vi "Teleop.vi"(0 "Call Context":T10) -> (6 "SubState 3":T1, 8 "SubState 4":T1, 9 "SubState 5":T9, 11 "Loop 3 Data":T5, 13 "Loop 4 Data":T4, 14 "SubState 0":T1=enum."driver control", 15 "Loop 1 Data":T7, 16 "Loop 0 Data":T8, 17 "SubState 1":T1, 18 "Loop 2 Data":T6, 19 "SubState 2":T1)   [LabVIEW 2013]
uses:
  typedefs/subStates.ctl
  <vilib>/Rock Robotics/WPI/DriverStation/WPI_DriverStationDerivedRobotMode.ctl
  typedefs/singleUseSubstate.ctl
  typedefs/Loop Datatypes/Loop 0 Datatype.ctl
  typedefs/Loop Datatypes/Loop 1 Datatype.ctl
  typedefs/Loop Datatypes/Loop 2 Datatype.ctl
  typedefs/Loop Datatypes/Loop 3 Datatype.ctl
  typedefs/Loop Datatypes/Loop 4 Datatype.ctl
  <vilib>/Rock Robotics/WPI/Joystick/WPI_JoystickDevRef.ctl
  <vilib>/Rock Robotics/WPI/Joystick/WPI_JoystickDeviceEnum.ctl
  typedefs/fg_typedef.ctl
  typedefs/vision enable.ctl
  <vilib>/Rock Robotics/WPI/Joystick/WPI_JoystickGetSetRefNum.vi
panel:
  out "prev lock state":T1
  out "JS3":T2
  out "Drive to DC":bool
  out "JS1":T2
  out "JS2":T2
  out "Exit Value":i32=-1
  # "Loop Data and Substates"
  # "Latch Loop"
  # "Drive Loop"
  # "Shooter Pneumatics Loop"
  # "Pickup/Passing Belts Loop"
  # "Pickup Arm Loop"
  # "Shifter Loop"
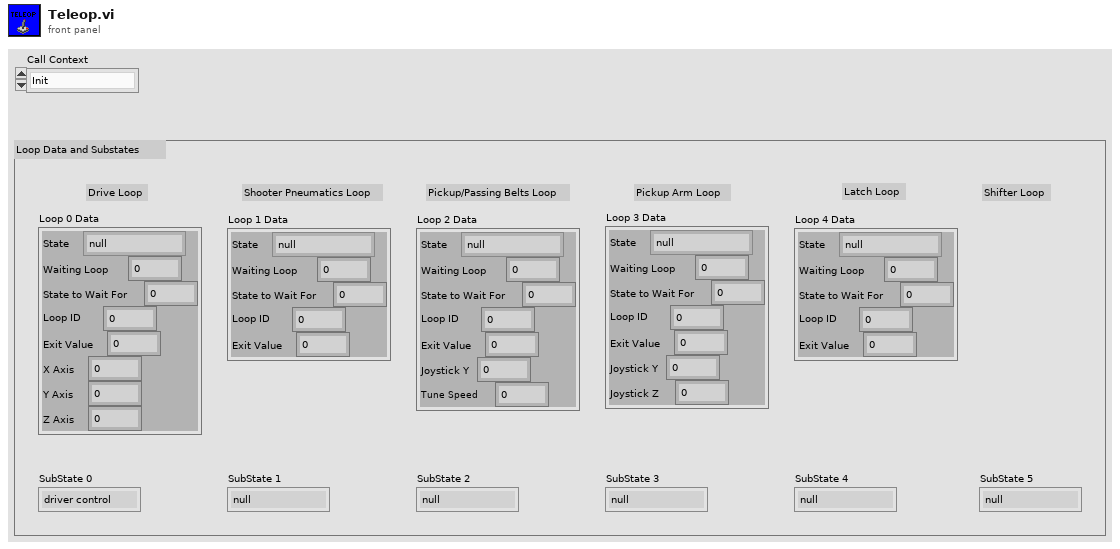
[diagram p1: front panel]
types:
  T1 = typedef "subStates.ctl" = enum16{"null", "wait", "driver control", "auto", "manual override", "hold position", "rotate", "pickup", "pass", "load", "goto shoot", "shoot", "cancel", "end"}
  T2 = typedef "WPI_JoystickDevRef.ctl" = cluster{"Device":T3}
  T3 = typedef "WPI_JoystickDeviceEnum.ctl" = enum16{"USB 1", "USB 2", "USB 3", "USB 4", "Kinect 1", "Kinect 2"}
  T4 = typedef "Loop 4 Datatype.ctl" = cluster{"State":T1, "Waiting Loop":i32, "State to Wait For":i32, "Loop ID":i32, "Exit Value":i32}
  T5 = typedef "Loop 3 Datatype.ctl" = cluster{"State":T1, "Waiting Loop":i32, "State to Wait For":i32, "Loop ID":i32, "Exit Value":i32, "Joystick Y":dbl, "Joystick Z":dbl}
  T6 = typedef "Loop 2 Datatype.ctl" = cluster{"State":T1, "Waiting Loop":i32, "State to Wait For":i32, "Loop ID":i32, "Exit Value":i32, "Joystick Y":dbl, "Tune Speed":dbl}
  T7 = typedef "Loop 1 Datatype.ctl" = cluster{"State":T1, "Waiting Loop":i32, "State to Wait For":i32, "Loop ID":i32, "Exit Value":i32}
  T8 = typedef "Loop 0 Datatype.ctl" = cluster{"State":T1, "Waiting Loop":i32, "State to Wait For":i32, "Loop ID":i32, "Exit Value":i32, "X Axis":dbl, "Y Axis":dbl, "Z Axis":dbl}
  T9 = typedef "singleUseSubstate.ctl" = enum16{"null", "wait", "shift high", "shift low", "extend shooter", "retract shooter", "close latch", "open latch"}
  T10 = typedef "WPI_DriverStationDerivedRobotMode.ctl" = enum16{"Init", "Execute", "Stop"}
  T11 = cluster{"axis 1 (x)":dbl, "axis 2 (y)":dbl, "axis 3 (throttle)":dbl, "axis 4":dbl, "axis 5":dbl, "axis 6":dbl}
  T12 = typedef "WPI_EncoderDevRef.ctl" = cluster{"DevStatus":errorcluster, "EncoderIndex":T13, "CounterIndex":T14, "DistancePerCount":dbl, "Decoding Type":T15}
  T13 = typedef "FPGA_EncoderIdx.ctl" = enum8{"Enc 0", "Enc 1", "Enc 2", "Enc 3", "Invalid"}
  T14 = typedef "FPGA_CounterCtrSystemIndex.ctl" = enum8{"Ctr 0", "Ctr 1", "Ctr 2", "Ctr 3", "Ctr 4", "Ctr 5", "Ctr 6", "Ctr 7", "Invalid"}
  T15 = typedef "WPI_EncoderType.ctl" = enum16{"1x", "2x", "4x"}
  T16 = typedef "vision enable.ctl" = enum16{"Enable", "Disable", "Stop"}
  T17 = typedef "fg_typedef.ctl" = enum16{"Get", "Set"}
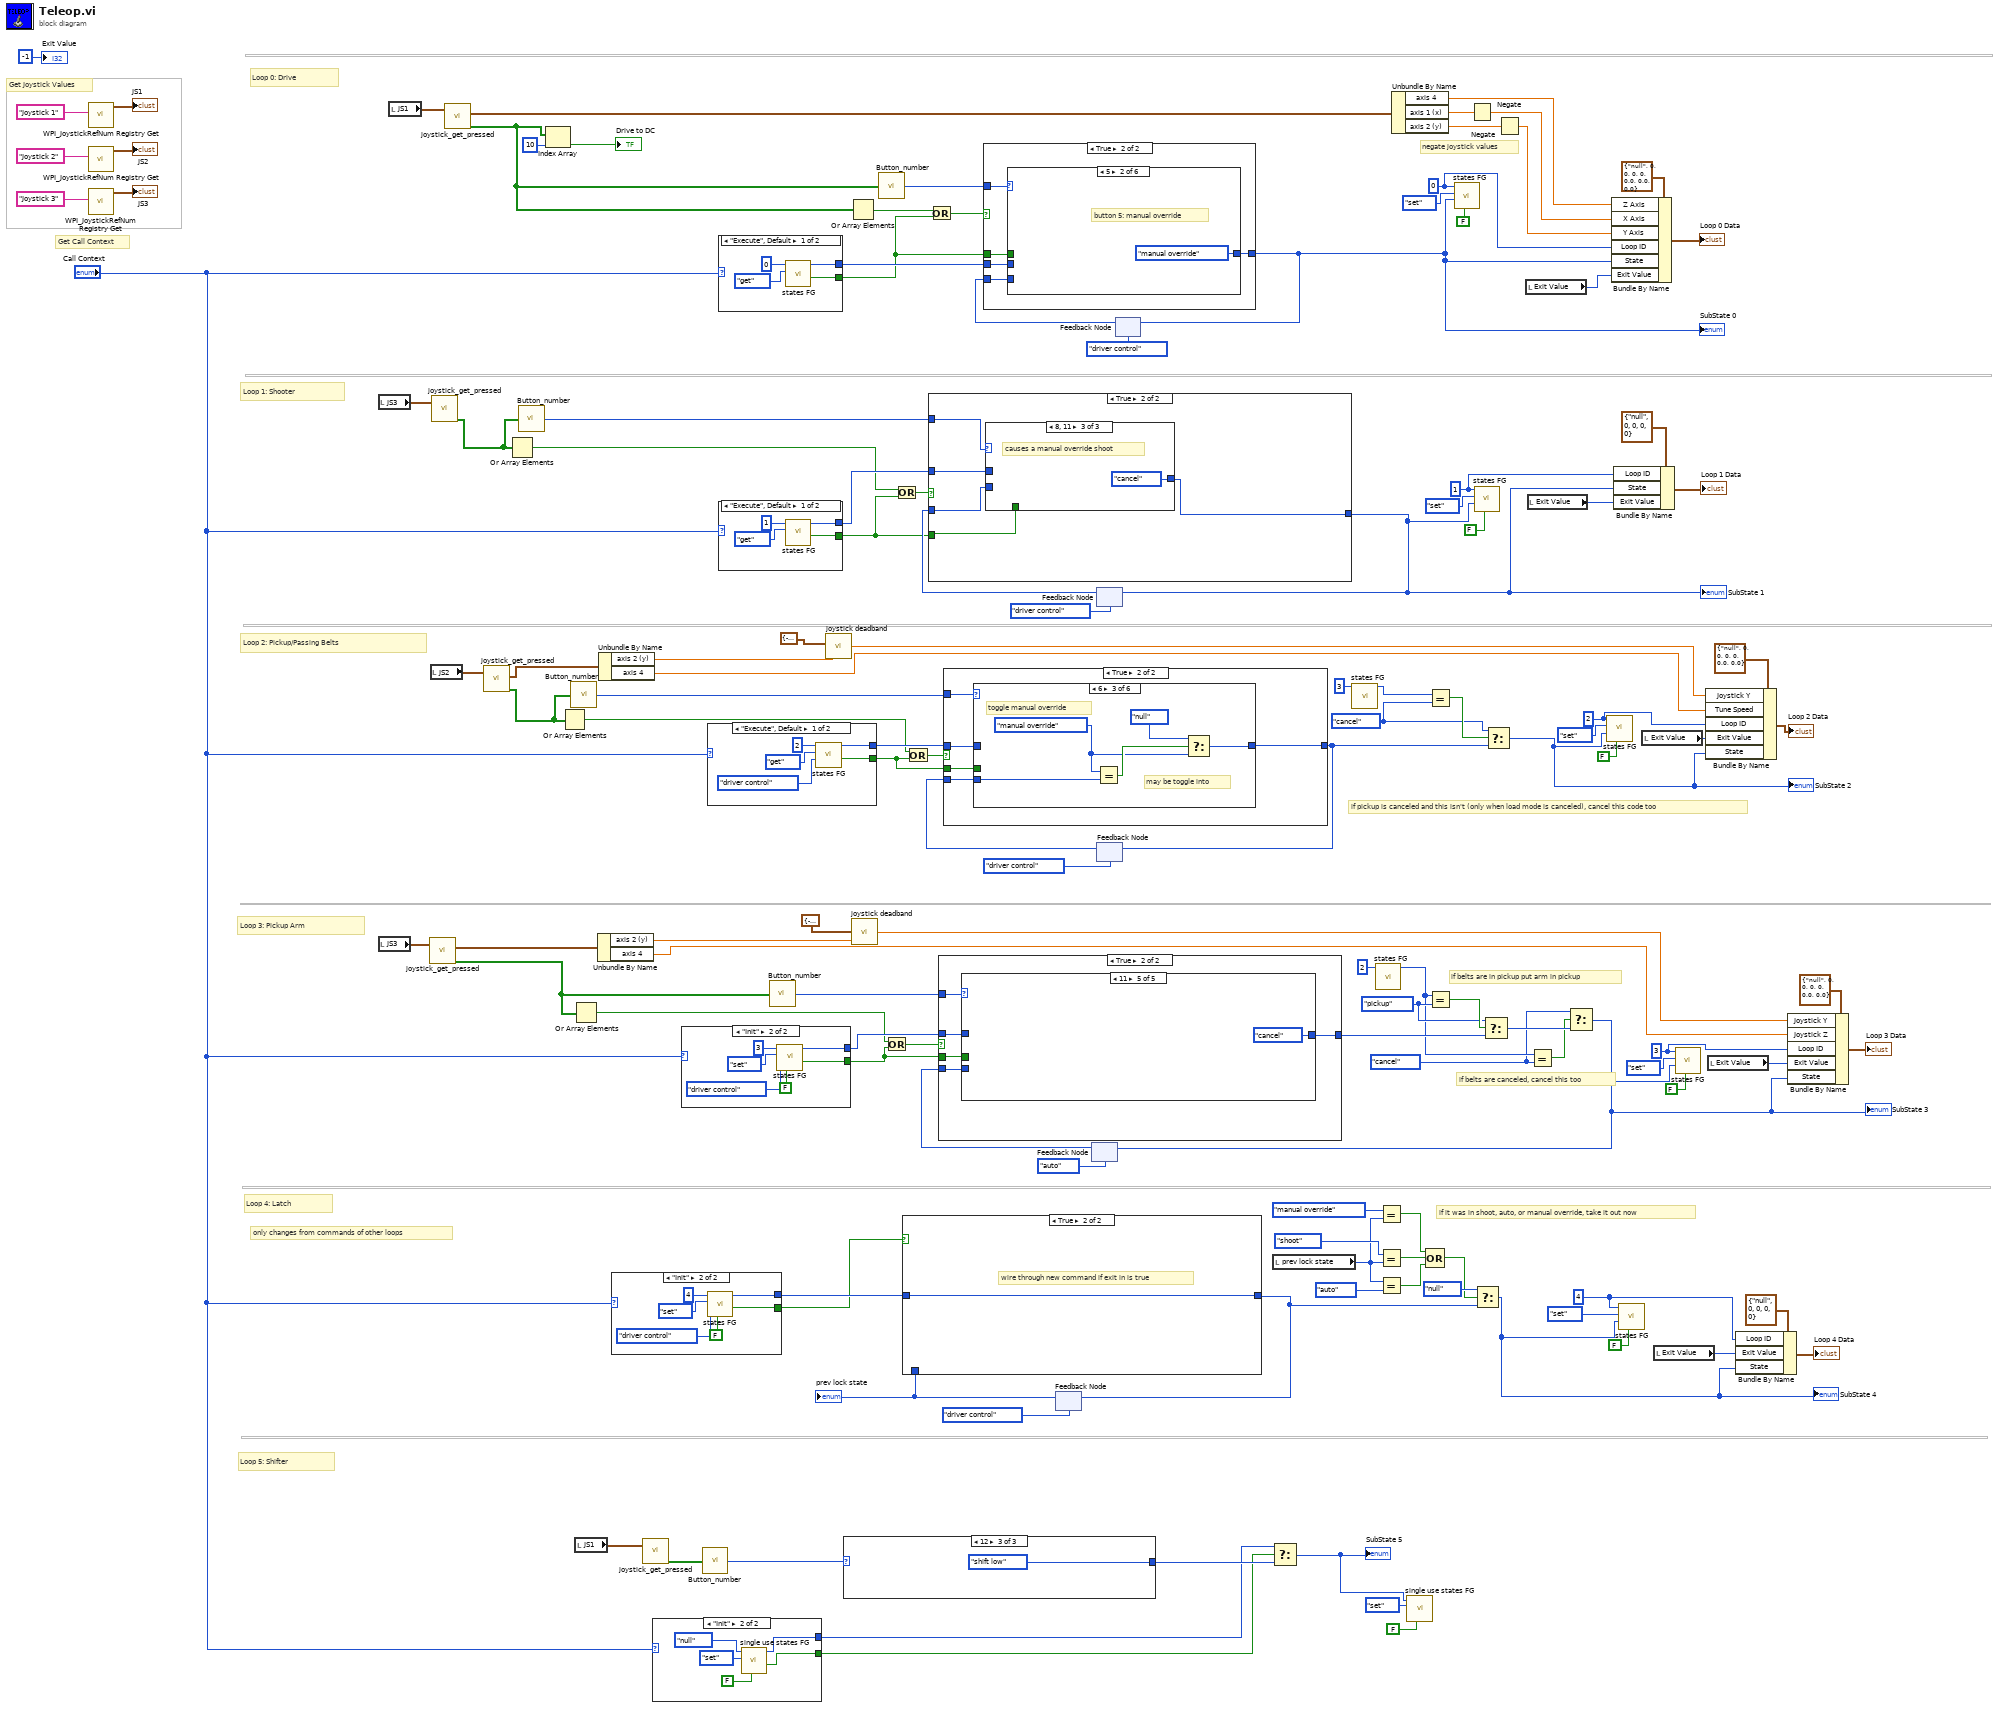
[diagram p0: block diagram]
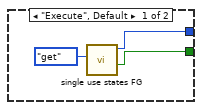
[diagram p2: hidden frame]
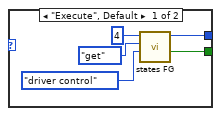
[diagram p4: hidden frame]
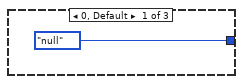
[diagram p5: hidden frame]
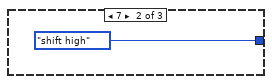
[diagram p6: hidden frame]
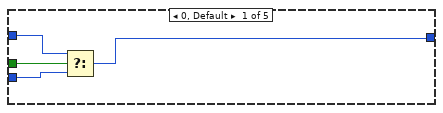
[diagram p8: hidden frame]
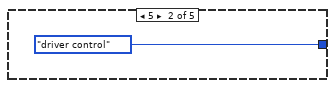
[diagram p9: hidden frame]
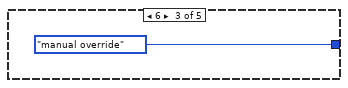
[diagram p10: hidden frame]
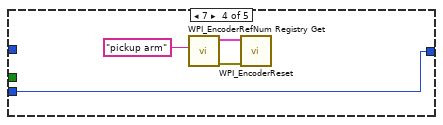
[diagram p11: hidden frame]
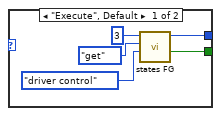
[diagram p12: hidden frame]
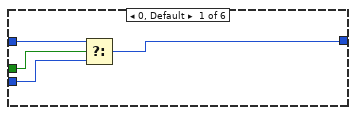
[diagram p14: hidden frame]
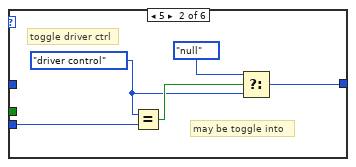
[diagram p15: hidden frame]
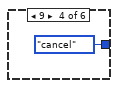
[diagram p16: hidden frame]
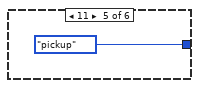
[diagram p17: hidden frame]
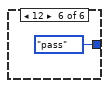
[diagram p18: hidden frame]
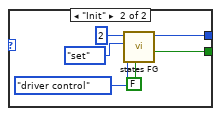
[diagram p19: hidden frame]
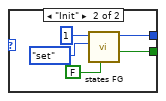
[diagram p20: hidden frame]
diagram:
  w7 = subStates."cancel" ("y")
  w14 = subStates."cancel" ("y")
  w31 = subStates."pickup" ("y")
  w42 = 4 ("Loop ID")
  w105 = 3 ("Loop ID")
  w106 = 2 ("Loop ID")
  w115 = 1 ("Loop ID")
  w117 = 0 ("Loop ID")
  # "if pickup is canceled and this isn't (only when load mode is canceled), cancel this code too"
  # "if belts are canceled, cancel this too"
  # "only changes from commands of other loops"
  # "if it was in shoot, auto, or manual override, take it out now"
  # "if belts are in pickup put arm in pickup"
  # "negate joystick values"
  # "Get Call Context"
  # "Get Joystick Values"
  # "Loop 4: Latch"
  # "Loop 3: Pickup Arm"
  # "Loop 5: Shifter"
  # "Loop 2: Pickup/Passing Belts"
  # "Loop 1: Shooter"
  # "Loop 0: Drive"
  n1 = call <vilib>:"WPI_JoystickRefNum Registry Get.vi"("refnum name"="Joystick 1") -> ("JoystickDevRef"=→"JS1":T2)  [unwired: 9 in, 1 out]
  n2 = call <vilib>:"WPI_JoystickRefNum Registry Get.vi"("refnum name"="Joystick 2") -> ("JoystickDevRef"=→"JS2":T2)  [unwired: 9 in, 1 out]
  n3 = call <vilib>:"WPI_JoystickRefNum Registry Get.vi"("refnum name"="Joystick 3") -> ("JoystickDevRef"=→"JS3":T2)  [unwired: 9 in, 1 out]
  n4 = local read "JS3"() -> (w82:T2)
  n5 = local read "JS3"() -> (w67:T2)
  n6 = local read "JS1"() -> (w83:T2)
  n7 = call "joystick_get_pressed.vi"("JoystickDevRef 2"=w67) -> ("Axes"=w71:T11, "Buttons Pressed?"=w49:bool[])  [unwired: 1 in, 2 out]
  n8 = local read "JS2"() -> (w56:T2)
  n9 = call "joystick_get_pressed.vi"("JoystickDevRef 2"=w82) -> ("Buttons Pressed?"=w51:bool[])  [unwired: 1 in, 3 out]
  n10 = call "joystick_get_pressed.vi"("JoystickDevRef 2"=w83) -> ("Axes"=w87:T11, "Buttons Pressed?"=w63:bool[])  [unwired: 1 in, 2 out]
  n11 = call "joystick_get_pressed.vi"("JoystickDevRef 2"=w56) -> ("Axes"=w39:T11, "Buttons Pressed?"=w40:bool[])  [unwired: 1 in, 2 out]
  n12 = Or Array Elements(Boolean array=w51) -> (logical OR=w74:bool)
  n13 = call "Button_number.vi"("Button Array"=w51) -> ("Button Pressed"=w76:i32)
  n14 = Index Array(array=w63, index=10) -> (element=→"Drive to DC":bool)
  n15 = Or Array Elements(Boolean array=w40) -> (logical OR=w55:bool)
  n16 = call "Button_number.vi"("Button Array"=w40) -> ("Button Pressed"=w54:i32)
  n17 = Or Array Elements(Boolean array=w49) -> (logical OR=w70:bool)
  n18 = local read "JS1"() -> (w59:T2)
  n19 = Unbundle By Name(w71) -> ("axis 2 (y)"=w66:dbl, "axis 4"=w35:dbl)
  n20 = Unbundle By Name(w39) -> ("axis 2 (y)"=w48:dbl, "axis 4"=w37:dbl)
  n21 = case shown="\"Init\"" "Call Context" {
    tunnel: [w136 w142] -> w19
    tunnel: [w134 w139] -> w44
    frame "Execute", Default {
      n22 = call "states FG.vi"("subState in"=subStates."driver control", "menu (get)"=enum16{"set", "get"}."get", "Loop ID"=4) -> ("exit out"=w136:bool, "subState out"=w134:T1)  [unwired: 5 in, 2 out]
    }
    frame "Init" {
      n23 = call "states FG.vi"("exit in"=FALSE, "subState in"=subStates."driver control", "menu (get)"=enum16{"set", "get"}."set", "Loop ID"=4) -> ("exit out"=w142:bool, "subState out"=w139:T1)  [unwired: 4 in, 2 out]
    }
  }
  n24 = call "joystick_get_pressed.vi"("JoystickDevRef 2"=w59) -> ("Buttons Pressed?"=w61:bool[])  [unwired: 1 in, 3 out]
  n25 = case shown="\"Init\"" "Call Context" {
    tunnel: [w146 w148] -> w4
    tunnel: [w145 w149] -> w5
    frame "Execute", Default {
      n26 = call "single use states FG.vi"("menu (get)"=enum16{"set", "get"}."get") -> ("exit out"=w146:bool, "substate out"=w145:T9)  [unwired: 7 in, 2 out]
    }
    frame "Init" {
      n27 = call "single use states FG.vi"("exit in"=FALSE, "menu (get)"=enum16{"set", "get"}."set", "substate"=singleUseSubstate."null") -> ("exit out"=w148:bool, "substate out"=w149:T9)  [unwired: 5 in, 2 out]
    }
  }
  n28 = case shown="\"Init\"" "Call Context" {
    tunnel: [w155 w161] -> w68
    tunnel: [w153 w158] -> w103
    frame "Execute", Default {
      n29 = call "states FG.vi"("subState in"=subStates."driver control", "menu (get)"=enum16{"set", "get"}."get", "Loop ID"=3) -> ("exit out"=w155:bool, "subState out"=w153:T1)  [unwired: 5 in, 2 out]
    }
    frame "Init" {
      n30 = call "states FG.vi"("exit in"=FALSE, "subState in"=subStates."driver control", "menu (get)"=enum16{"set", "get"}."set", "Loop ID"=3) -> ("exit out"=w161:bool, "subState out"=w158:T1)  [unwired: 4 in, 2 out]
    }
  }
  n31 = call "Button_number.vi"("Button Array"=w61) -> ("Button Pressed"=w60:i32)
  n32 = case shown="\"Execute\", Default" "Call Context" {
    tunnel: [w166 w172] -> w73
    tunnel: [w164 w169] -> w122
    frame "Execute", Default {
      n33 = call "states FG.vi"("subState in"=subStates."driver control", "menu (get)"=enum16{"set", "get"}."get", "Loop ID"=2) -> ("exit out"=w166:bool, "subState out"=w164:T1)  [unwired: 5 in, 2 out]
    }
    frame "Init" {
      n34 = call "states FG.vi"("exit in"=FALSE, "subState in"=subStates."driver control", "menu (get)"=enum16{"set", "get"}."set", "Loop ID"=2) -> ("exit out"=w172:bool, "subState out"=w169:T1)  [unwired: 4 in, 2 out]
    }
  }
  n35 = case shown="\"Execute\", Default" "Call Context" {
    tunnel: [w176 w181] -> w80
    tunnel: [w175 w179] -> w120
    frame "Execute", Default {
      n36 = call "states FG.vi"("menu (get)"=enum16{"set", "get"}."get", "Loop ID"=0) -> ("exit out"=w176:bool, "subState out"=w175:T1)  [unwired: 6 in, 2 out]
    }
    frame "Init" {
      n37 = call "states FG.vi"("exit in"=FALSE, "menu (get)"=enum16{"set", "get"}."set", "Loop ID"=0) -> ("exit out"=w181:bool, "subState out"=w179:T1)  [unwired: 5 in, 2 out]
    }
  }
  n38 = case shown="\"Execute\", Default" "Call Context" {
    tunnel: [w185 w190] -> w77
    tunnel: [w184 w188] -> w119
    frame "Execute", Default {
      n39 = call "states FG.vi"("menu (get)"=enum16{"set", "get"}."get", "Loop ID"=1) -> ("exit out"=w185:bool, "subState out"=w184:T1)  [unwired: 6 in, 2 out]
    }
    frame "Init" {
      n40 = call "states FG.vi"("exit in"=FALSE, "menu (get)"=enum16{"set", "get"}."set", "Loop ID"=1) -> ("exit out"=w190:bool, "subState out"=w188:T1)  [unwired: 5 in, 2 out]
    }
  }
  n41 = call "Button_number.vi"("Button Array"=w49) -> ("Button Pressed"=w69:i32)
  n42 = call "joystick deadband.vi"("Joystick In"=w48, "Deadband Range"=cluster{"Deadband Min":dbl, "Deadband Max":dbl} {"Deadband Min"=-0.05, "Deadband Max"=0.05}) -> ("Joystick Out"=w38:dbl)  [unwired: 4 in]
  n43 = case shown="12" w60 {
    tunnel: [singleUseSubstate."null" ("Enum") singleUseSubstate."shift high" ("Enum") singleUseSubstate."shift low" ("Enum")] -> w95
    frame 0, Default {
    }
    frame 7 {
    }
    frame 12 {
    }
  }
  n44 = Or Array Elements(Boolean array=w63) -> (logical OR=w81:bool)
  n45 = call "joystick deadband.vi"("Joystick In"=w66, "Deadband Range"=cluster{"Deadband Min":dbl, "Deadband Max":dbl} {"Deadband Min"=-0.05, "Deadband Max"=0.05}) -> ("Joystick Out"=w36:dbl)  [unwired: 4 in]
  n46 = call "Button_number.vi"("Button Array"=w63) -> ("Button Pressed"=w86:i32)
  n47 = Or(x=w70, y=w68) -> (x .or. y?=w72:bool)
  n48 = Or(x=w74, y=w77) -> (x .or. y?=w78:bool)
  n49 = Or(x=w55, y=w73) -> (x .or. y?=w75:bool)
  n50 = Or(x=w81, y=w80) -> (x .or. y?=w79:bool)
  n51 = feedback #1(subStates."driver control" ("Drive SubState")) -> (w18:T1)
  "prev lock state" <- w18
  n52 = case shown="True" w19 {
    tunnel: [w196 w197] -> w29
    tunnel: w44 -> [_ w197]
    tunnel: w18 -> [w196 _]
    frame False {
      # "*yawn* nothing to do...wire through the previous state"
    }
    frame True {
      # "wire through new command if exit in is true"
    }
  }
  n53 = feedback-in #1(w29) -> ()
  n54 = feedback #2(subStates."auto" ("Drive SubState")) -> (w100:T1)
  n55 = case shown="True" w72 {
    tunnel: w100 -> [w198 w199]
    tunnel: [w198 w200] -> w33
    tunnel: w103 -> [_ w201]
    tunnel: w69 -> [_ w203]
    tunnel: w68 -> [_ w202]
    frame False {
      # "boring drivers, not pressing anything...wire through the previous state"
    }
    frame True {
      n56 = case shown="11" w203 {
        tunnel: w202 -> [w207 _ _ _ _]
        tunnel: w199 -> [w206 _ _ w213 _]
        tunnel: w201 -> [w205 _ _ _ _]
        tunnel: [w204 subStates."driver control" ("Drive SubState") subStates."manual override" ("Drive SubState") w213 subStates."cancel" ("Drive SubState")] -> w200
        frame 0, Default {
          n57 = Select(t=w205, s=w207, f=w206) -> (s? t:f=w204:T1)
        }
        frame 5 {
        }
        frame 6 {
        }
        frame 7 {
          n58 = call <vilib>:"WPI_EncoderRefNum Registry Get.vi"("refnum name"="pickup arm") -> ("error out"=w211:errorcluster, "EncoderDevRef"=w210:T12)  [unwired: 9 in]
          n59 = call <vilib>:"WPI_EncoderReset.vi"("error in (no error)"=w211, "EncoderDevRef"=w210) -> ()  [unwired: 8 in, 2 out]
        }
        frame 11 {
        }
      }
    }
  }
  n60 = feedback #3(subStates."driver control" ("Drive SubState")) -> (w121:T1)
  n61 = case shown="True" w78 {
    tunnel: w121 -> [w215 w219]
    tunnel: [w215 w216] -> w88
    tunnel: w119 -> [_ w220]
    tunnel: w76 -> [_ w218]
    tunnel: w77 -> [_ w217]
    frame False {
      # "nothing pressed here, move along (wire through the previous state)"
    }
    frame True {
      n62 = case shown="8, 11" w218 {
        tunnel: w220 -> [w223 _ _]
        tunnel: w219 -> [w222 _ _]
        tunnel: [w221 subStates."load" ("Drive SubState") subStates."cancel" ("Drive SubState")] -> w216
        tunnel: w217 -> [w224 _ _]
        frame 0, Default {
          n63 = Select(t=w223, s=w224, f=w222) -> (s? t:f=w221:T1)
        }
        frame 2 {
        }
        frame 8, 11 {
          # "causes a manual override shoot"
        }
      }
    }
  }
  "SubState 1" <- w88
  n64 = feedback-in #3(w88) -> ()
  n65 = feedback #4(subStates."driver control" ("Drive SubState")) -> (w125:T1)
  n66 = case shown="True" w75 {
    tunnel: w125 -> [w227 w229]
    tunnel: [w227 w228] -> w10
    tunnel: w122 -> [_ w230]
    tunnel: w54 -> [_ w232]
    tunnel: w73 -> [_ w231]
    frame False {
      # "nothing pressed here, move along obviously and wire through the previous state"
    }
    frame True {
      n67 = case shown="6" w232 {
        tunnel: w231 -> [w236 _ _ _ _ _]
        tunnel: w230 -> [w235 _ _ _ _ _]
        tunnel: w229 -> [w234 w241 w243 _ _ _]
        tunnel: [w233 w237 w242 subStates."cancel" ("Drive SubState") subStates."pickup" ("Drive SubState") subStates."pass" ("Drive SubState")] -> w228
        frame 0, Default {
          n68 = Select(t=w235, s=w236, f=w234) -> (s? t:f=w233:T1)
        }
        frame 5 {
          w239 = subStates."driver control" ("Drive SubState")
          # "may be toggle into"
          # "toggle driver ctrl"
          n69 = Equal?(x=w239, y=w241) -> (x = y?=w240:bool)
          n70 = Select(t=subStates."null", s=w240, f=w239) -> (s? t:f=w237:T1)
        }
        frame 6 {
          w244 = subStates."manual override" ("Drive SubState")
          # "may be toggle into"
          # "toggle manual override"
          n71 = Equal?(x=w244, y=w243) -> (x = y?=w246:bool)
          n72 = Select(t=subStates."null", s=w246, f=w244) -> (s? t:f=w242:T1)
        }
        frame 9 {
        }
        frame 11 {
        }
        frame 12 {
        }
      }
    }
  }
  n73 = feedback-in #4(w10) -> ()
  n74 = feedback #5(subStates."driver control" ("Drive SubState")) -> (w127:T1)
  n75 = case shown="True" w79 {
    tunnel: w127 -> [w250 w252]
    tunnel: [w250 w251] -> w58
    tunnel: w120 -> [_ w253]
    tunnel: w86 -> [_ w255]
    tunnel: w80 -> [_ w254]
    frame False {
      # "keep current state, no change necessary"
    }
    frame True {
      n76 = case shown="5" w255 {
        tunnel: w254 -> [w259 _ _ _ _ _]
        tunnel: w253 -> [w258 _ _ _ _ _]
        tunnel: w252 -> [w257 _ w265 w266 w274 _]
        tunnel: [w256 subStates."manual override" ("Drive SubState") w261 w266 w275 subStates."driver control" ("Drive SubState")] -> w251
        frame 0, Default {
          n77 = Select(t=w258, s=w259, f=w257) -> (s? t:f=w256:T1)
        }
        frame 5 {
          # "button 5: manual override"
        }
        frame 1 {
          w262 = subStates."hold position" ("x")
          # "button 1, hold position toggle"
          n78 = Equal?(x=w262, y=w265) -> (x = y?=w264:bool)
          n79 = Select(t=subStates."driver control" ("Drive SubState"), s=w264, f=w262) -> (s? t:f=w261:T1)
        }
        frame 8 {
          n80 = disable-structure shown="Enabled" {
            frame Disabled {
              w269 = vision_enable."Enable" ("y")
              # "toggle vision"
              n81 = call "vision_fg.vi"("Menu"=fg_typedef."Get") -> ("State Out"=w271:T16)  [unwired: 2 in, 1 out]
              n82 = Equal?(x=w271, y=w269) -> (x = y?=w270:bool)
              n83 = Select(t=vision_enable."Disable" ("y"), s=w270, f=w269) -> (s? t:f=w267:T16)
              n84 = call "vision_fg.vi"("Action"=w267, "Menu"=fg_typedef."Set") -> ()  [unwired: 1 in, 2 out]
            }
            frame Enabled {
              # "no vision at suffield"
            }
          }
        }
        frame 9 {
          n85 = disable-structure shown="Enabled" {
            disable-tunnel: [subStates."goto shoot" ("Drive SubState") w279] -> w275
            disable-tunnel: w274 -> [_ w279]
            frame Disabled {
              # "go to shoot location"
              n86 = call "vision_fg.vi"("Action"=vision_enable."Enable", "Menu"=fg_typedef."Set") -> ()  [unwired: 1 in, 2 out]
            }
            frame Enabled {
              # "no vision at suffield"
            }
          }
        }
        frame 11 {
          # "put robot drive in driver control"
          n87 = call "vision_fg.vi"("Action"=vision_enable."Disable", "Menu"=fg_typedef."Set") -> ()  [unwired: 1 in, 2 out]
        }
      }
    }
  }
  "SubState 0" <- w58
  n88 = feedback-in #5(w58) -> ()
  n89 = Select(t=w5, s=w4, f=w95) -> (s? t:f=w2:T9)
  "SubState 5" <- w2
  n90 = local read "prev lock state"() -> (w25:T1)
  n91 = call "states FG.vi"("Loop ID"=3) -> ("subState out"=w11:T1)  [unwired: 7 in, 3 out]
  n92 = call "states FG.vi"("Loop ID"=2) -> ("subState out"=w17:T1)  [unwired: 7 in, 3 out]
  n93 = Equal?(x=subStates."manual override", y=w25) -> (x = y?=w23:bool)
  n94 = Equal?(x=subStates."shoot", y=w25) -> (x = y?=w22:bool)
  n95 = Equal?(x=w25, y=subStates."auto") -> (x = y?=w21:bool)
  n96 = Unbundle By Name(w87) -> ("axis 4"=w64:dbl, "axis 1 (x)"=w92:dbl, "axis 2 (y)"=w91:dbl)
  n97 = call "single use states FG.vi"("exit in"=FALSE, "menu (get)"=enum16{"set", "get"}."set", "substate"=w2) -> ()  [unwired: 5 in, 4 out]
  n98 = Compound Arithmetic op=OR(w23, w22, w21) -> (w20:bool)
  n99 = Equal?(x=w11, y=w7) -> (x = y?=w9:bool)
  n100 = Equal?(x=w17, y=w31) -> (x = y?=w32:bool)
  n101 = call "states FG.vi"("exit in"=FALSE, "subState in"=w58, "menu (get)"=enum16{"set", "get"}."set", "Loop ID"=w117) -> ()  [unwired: 4 in, 4 out]
  n102 = Negate(x=w92) -> (-x=w90:dbl)
  n103 = call "states FG.vi"("exit in"=FALSE, "subState in"=w88, "menu (get)"=enum16{"set", "get"}."set", "Loop ID"=w115) -> ()  [unwired: 4 in, 4 out]
  n104 = Select(t=subStates."null", s=w20, f=w29) -> (s? t:f=w28:T1)
  "SubState 4" <- w28
  n105 = Select(t=w31, s=w32, f=w33) -> (s? t:f=w16:T1)
  n106 = Select(t=w7, s=w9, f=w10) -> (s? t:f=w8:T1)
  "SubState 2" <- w8
  n107 = Negate(x=w91) -> (-x=w89:dbl)
  n108 = local read "Exit Value"() -> (w113:i32)
  n109 = local read "Exit Value"() -> (w112:i32)
  n110 = Equal?(x=w17, y=w14) -> (x = y?=w15:bool)
  n111 = Select(t=w14, s=w15, f=w16) -> (s? t:f=w13:T1)
  "SubState 3" <- w13
  n112 = feedback-in #2(w13) -> ()
  n113 = call "states FG.vi"("exit in"=FALSE, "subState in"=w8, "menu (get)"=enum16{"set", "get"}."set", "Loop ID"=w106) -> ()  [unwired: 4 in, 4 out]
  n114 = Bundle By Name(cluster=T8 {"State"=enum."null", "Waiting Loop"=0, "State to Wait For"=0, "Loop ID"=0, "Exit Value"=0, "X Axis"=0.0, "Y Axis"=0.0, "Z Axis"=0.0} ("Cluster"), "Z Axis"=w64, "X Axis"=w90, "Y Axis"=w89, "Loop ID"=w117, "State"=w58, "Exit Value"=w113) -> (→"Loop 0 Data":T8)
  n115 = Bundle By Name(cluster=T7 {"State"=enum."null", "Waiting Loop"=0, "State to Wait For"=0, "Loop ID"=0, "Exit Value"=0} ("Cluster"), "Loop ID"=w115, "State"=w88, "Exit Value"=w112) -> (→"Loop 1 Data":T7)
  n116 = call "states FG.vi"("exit in"=FALSE, "subState in"=w28, "menu (get)"=enum16{"set", "get"}."set", "Loop ID"=w42) -> ()  [unwired: 4 in, 4 out]
  n117 = local read "Exit Value"() -> (w107:i32)
  n118 = local read "Exit Value"() -> (w43:i32)
  n119 = call "states FG.vi"("exit in"=FALSE, "subState in"=w13, "menu (get)"=enum16{"set", "get"}."set", "Loop ID"=w105) -> ()  [unwired: 4 in, 4 out]
  n120 = Bundle By Name(cluster=T6 {"State"=enum."null", "Waiting Loop"=0, "State to Wait For"=0, "Loop ID"=0, "Exit Value"=0, "Joystick Y"=0.0, "Tune Speed"=0.0} ("Loop 2 Data"), "Joystick Y"=w38, "Tune Speed"=w37, "Loop ID"=w106, "Exit Value"=w107, "State"=w8) -> (→"Loop 2 Data":T6)
  n121 = local read "Exit Value"() -> (w104:i32)
  n122 = Bundle By Name(cluster=T4 {"State"=enum."null", "Waiting Loop"=0, "State to Wait For"=0, "Loop ID"=0, "Exit Value"=0} ("Loop 4 Data"), "Loop ID"=w42, "Exit Value"=w43, "State"=w28) -> (→"Loop 4 Data":T4)
  n123 = Bundle By Name(cluster=T5 {"State"=enum."null", "Waiting Loop"=0, "State to Wait For"=0, "Loop ID"=0, "Exit Value"=0, "Joystick Y"=0.0, "Joystick Z"=0.0} ("Loop 3 Data"), "Joystick Y"=w36, "Joystick Z"=w35, "Loop ID"=w105, "Exit Value"=w104, "State"=w13) -> (→"Loop 3 Data":T5)
  "Exit Value" <- -1 ("Exit Value")
